vi "XML Script - Tag Strings.vi"(0 "XML Script Tag":T1=enum."Control") -> (2 "XML String - Begin Tag":string, 3 "XML String - End Tag":string)   [LabVIEW 2017]
uses:
  <vilib>/_script/XML Scripting/XML Script Tag.ctl
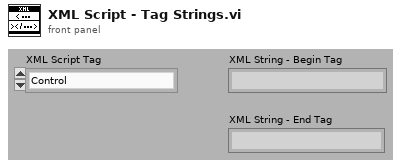
[diagram p1: front panel]
types:
  T1 = typedef "XML Script Tag.ctl" = enum16{"Script", "Function", "SubVI", "GrowableFunction", "Structure", "MultiframeStructure", "Frame", "Tunnel", "ShiftRegister", "Constant", "Control", "Terminal", "Wire", "StaticVIReference", "ControlTerminal", "CompoundArithmetic", "FlatSequence", "FlatSequenceFrame", "MathScriptCallByRef", "BuildArray", "GenericSubVI", "MathScriptNode"}
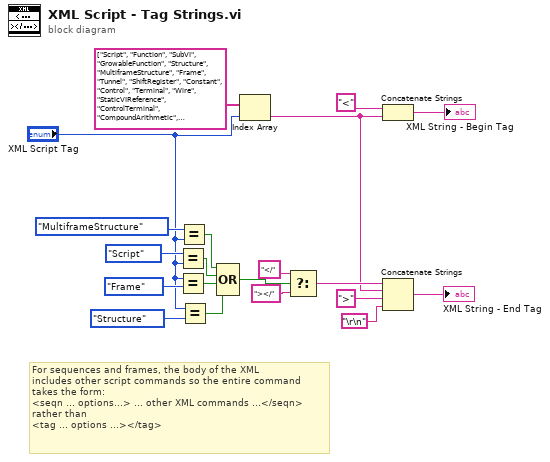
[diagram p0: block diagram]
diagram:
  # "For sequences and frames, the body of the XML\nincludes other script commands so the entire command\ntakes the form:\n<seqn ... options...> ... other XML commands ...</seqn>\nrather than\n<tag ... options ...></tag>"
  n1 = Equal?(x=XML_Script_Tag."Script", y="XML Script Tag") -> (x = y?=w4:bool)
  n2 = Equal?(x="XML Script Tag", y=XML_Script_Tag."Frame" ("XML Script Tag")) -> (x = y?=w10:bool)
  n3 = Equal?(x=XML_Script_Tag."MultiframeStructure" ("XML Script Tag"), y="XML Script Tag") -> (x = y?=w5:bool)
  n4 = Equal?(x="XML Script Tag", y=XML_Script_Tag."Structure" ("XML Script Tag")) -> (x = y?=w9:bool)
  n5 = Compound Arithmetic op=OR(w5, w4, w10, w9) -> (w14:bool)
  n6 = Index Array(array=string[] ["Script", "Function", "SubVI", "GrowableFunction", "Structure", "MultiframeStructure", "Frame", "Tunnel", "ShiftRegister", "Constant", "Control", "Terminal", "Wire", "StaticVIReference", "ControlTerminal", "CompoundArithmetic", "FlatSequence", "FlatSequenceFrame", "MathScriptCallByRef", "BuildArray", "GenericSubVI", "MathScriptNode"] ("Strings []"), index="XML Script Tag") -> (element=w1:string)
  n7 = Select(t="</", s=w14, f="></") -> (s? t:f=w11:string)
  n8 = Concatenate Strings("<", w1) -> (→"XML String - Begin Tag":string)
  n9 = Concatenate Strings(w11, w1, ">", "\r\n") -> (→"XML String - End Tag":string)
